vi "Data Viewer.vi"(8 "error in (no error)":errorcluster, 10 "stop pointer":refnum<class "Pointer.lvclass">, 11 "Server IP Address":string="localhost") -> (0 "error out":errorcluster)   [LabVIEW 2017, in "Data Viewer.lvlib"]
uses:
  Core/VIs/Data Viewer/Source/Data Viewer.lvlib
  <vilib>/NI/Memory Manager/Classes/Pointer/Pointer.lvclass
  Main VI/Application Data.ctl
  Buffer Reader/Queue Data.ctl
  Buffer Reader/Buffer Data.ctl
  Core/Classes/Configuration/Core/Transfer/Channel Configuration.ctl
  Core/Typedefs/Core Channel Configuration.ctl
  Core/Typedefs/DSF Data Type.ctl
  Core/Typedefs/DSF Settings Info.ctl
  Core/Typedefs/DSF Byte Order.ctl
  Core/Classes/Thread/Data Server/DSF Buffer Subset Descriptor.ctl
  Core/Typedefs/DSF Buffer Type.ctl
  Main VI/Values Channels.ctl
  Core/Classes/Configuration/Core/Framework/Framework Configuration.lvclass
  <vilib>/NI/Memory Manager/Classes/Pointer/Pointer.lvclass/Pointer.ctl
  <vilib>/NI/Memory Manager/Classes/Pointer/Write Bool.vi
  <vilib>/NI/Memory Manager/Classes/Pointer/Read Bool.vi
  <vilib>/NI/Memory Manager/Classes/Pointer/Get Address.vi
  <vilib>/NI/Memory Manager/Classes/Pointer/Set Address.vi
  <vilib>/NI/Memory Manager/Classes/Pointer/Set Size.vi
  <vilib>/NI/Memory Manager/Classes/Pointer/Set Internal.vi
  <vilib>/NI/Memory Manager/Classes/Pointer/Write (No Check).vi
  <vilib>/NI/Memory Manager/Classes/Pointer/Write (No Check) Bool.vi
  <vilib>/NI/Memory Manager/Classes/Pointer/Check Move.vi
  <vilib>/NI/Memory Manager/Classes/Pointer/Read (No Check).vi
  <vilib>/NI/Memory Manager/Classes/Pointer/Read (No Check) Bool.vi
  <vilib>/NI/Memory Manager/Classes/Pointer/Check Null Pointer.vi
  <vilib>/NI/Memory Manager/Classes/Pointer/Check Count.vi
  <vilib>/NI/Memory Manager/Classes/Pointer/Check Bounds (Power of 2).vi
  <vilib>/NI/Memory Manager/Classes/Pointer/Errors.vi
  <vilib>/NI/Memory Manager/Classes/Pointer/Null Pointer.vi
  <vilib>/NI/Memory Manager/Classes/Pointer/Get Size.vi
  <vilib>/NI/Memory Manager/Classes/Pointer/Out of Bounds.vi
  <vilib>/NI/Memory Manager/Classes/Pointer/Check Bounds.vi
  <vilib>/NI/Memory Manager/Classes/Pointer/Create Error.vi
  <vilib>/NI/Memory Manager/VIs/Write String to Source.vi
  <vilib>/NI/Memory Manager/Classes/Pointer/Write Pointer Size to Error.vi
  <vilib>/NI/Memory Manager/VIs/Write Numeric to Source.vi
  <vilib>/NI/Memory Manager/VIs/Write Numeric Scalar to Source (Base10 U64).vi
  <vilib>/NI/Memory Manager/Classes/Pointer/Check Bounds (Pointer).vi
  <vilib>/NI/Memory Manager/Classes/Pointer/Check Bounds (Buffer).vi
  <vilib>/NI/Memory Manager/VIs/New Error Cluster.vi
  <vilib>/NI/Memory Manager/VIs/New Error Cluster (512B).vi
  <vilib>/NI/Memory Manager/VIs/Set Error Status.vi
  <vilib>/NI/Memory Manager/VIs/Set Error Code.vi
  <vilib>/NI/Memory Manager/VIs/Set Error Source.vi
  <vilib>/NI/Memory Manager/Constants/Constants.vi
  <vilib>/NI/Memory Manager/Constants/Library Name.vi
  <vilib>/NI/Memory Manager/Classes/Pointer/Pointer Error Info.vi
  <vilib>/NI/Memory Manager/Constants/Pointer Class Name.vi
  <vilib>/NI/Memory Manager/Classes/Pointer/Buffer Underflow.vi
  Core/DSF Core.lvlib
  Core/Classes/Configuration/Core/Channel/Channel Configuration.lvclass
  Core/Classes/Configuration/Core/Transfer/Transfer Configuration.lvclass
panel:
  in  "Connect":bool
  out "Connected":bool
  in  "Item Tree":string(tree)
  out "Duration":u64 format="%d µs"
  out "Values":string
  out "ASCII":string
  out "Late Count":u64
  out "Iteration":u64
  out "Frequency":dbl format="%.1fHz"
  out "Size":u64 format="%dB"
  out "Decimation":u64
  out "Throughput":dbl format="%_3pB/s"
  out "Hex":string
  # "Data Viewer"
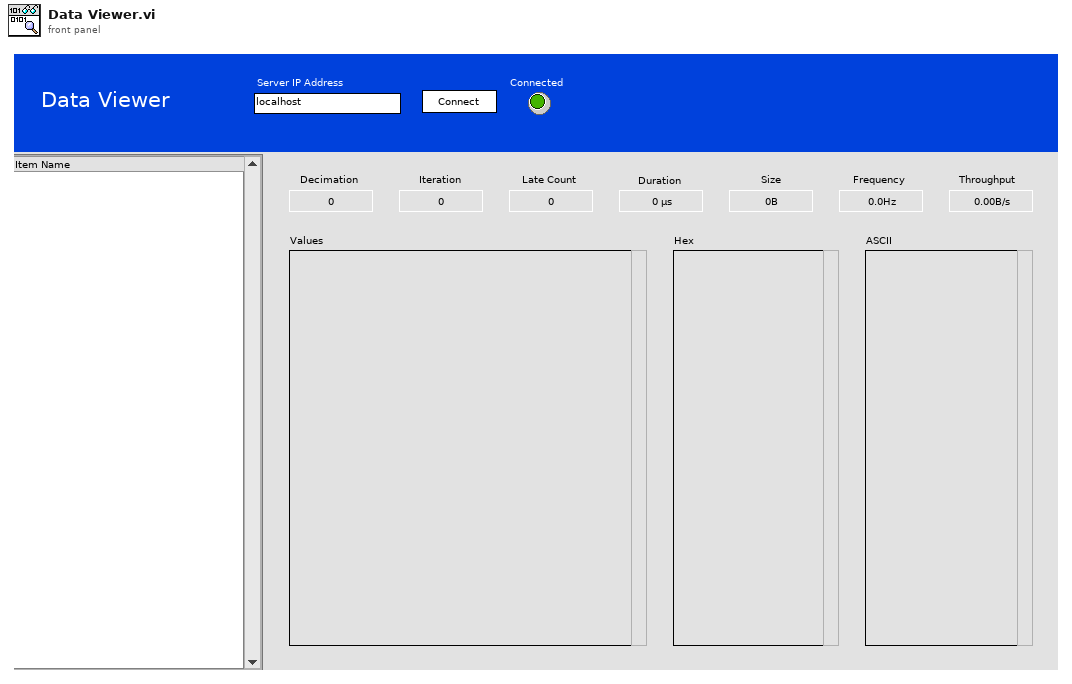
[diagram p1: front panel]
types:
  T1 = typedef "Data Viewer.lvlib/Queue Data.ctl" = cluster{"server ID":refnum<k5>, "Buffer data":T2}
  T2 = typedef "Data Viewer.lvlib/Buffer Data.ctl" = cluster{"decimation":u64, "avg bandwidth":dbl, "channels":T3[], "byte order":T7, "buffer descriptor":T8, "values channels":T10, "select start offset":u64, "select end offset":u64, "channel index":i32}
  T3 = typedef "DSF Core.lvlib/Transfer Configuration.lvclass/Channel Configuration.ctl" = cluster{"configuration":T4, "component settings":T6[]}
  T4 = typedef "DSF Core.lvlib/Channel Configuration.lvclass/Core Channel Configuration.ctl" = cluster{"name":string, "units":string, "engine data type":T5, "string data type":T5, "string offset":u64}
  T5 = typedef "DSF Core.lvlib/DSF Data Type.ctl" = enum8{"Bool", "SGL", "DBL", "I8", "I16", "I32", "I64", "U8", "U16", "U32", "U64"}
  T6 = typedef "DSF Core.lvlib/DSF Settings Info.ctl" = cluster{"component":string, "values":cluster{"key":string, "value":string}[]}
  T7 = typedef "DSF Core.lvlib/DSF Byte Order.ctl" = enum8{"big-endian", "little-endian"}
  T8 = typedef "DSF Core.lvlib/DSF Buffer Subset Descriptor.ctl" = cluster{"buffer type":T9, "plugin id":i32, "group id":i32, "transfer id":i32, "offset":u64, "length":i64}
  T9 = typedef "DSF Core.lvlib/DSF Buffer Type.ctl" = enum16{"Engine", "String"}
  T10 = typedef "Data Viewer.lvlib/Values Channels.ctl" = cluster{"index":i32, "count":i32, "engine offset":u64}
  T11 = typedef "Data Viewer.lvlib/Application Data.ctl" = cluster{"Item Tree Control":refnum<vi>, "Top-Level VI":refnum<vi>, "menu reference":refnum<k9>, "queue":refnum<queue>, "Stop Pointer":refnum<class "Pointer.lvclass">, "Buffer Variant":variant, "server ID":refnum<k5>, "framework tag":string, "Values":refnum<vi>, "Hex":refnum<vi>, "ASCII":refnum<vi>, "lines visible":i32, "values padding":i32, "current buffer data":T2, "Framework Configuration":refnum<class "Framework Configuration.lvclass">}
  T12 = typedef "LVPoint32TypeDef.ctl" = cluster{"Horizontal":i32, "Vertical":i32}
  T13 = typedef "DSF Core.lvlib/DSF Performance Metrics.ctl" = cluster{"framework period":u32, "iteration":u64, "late count":u64, "duration":u64}
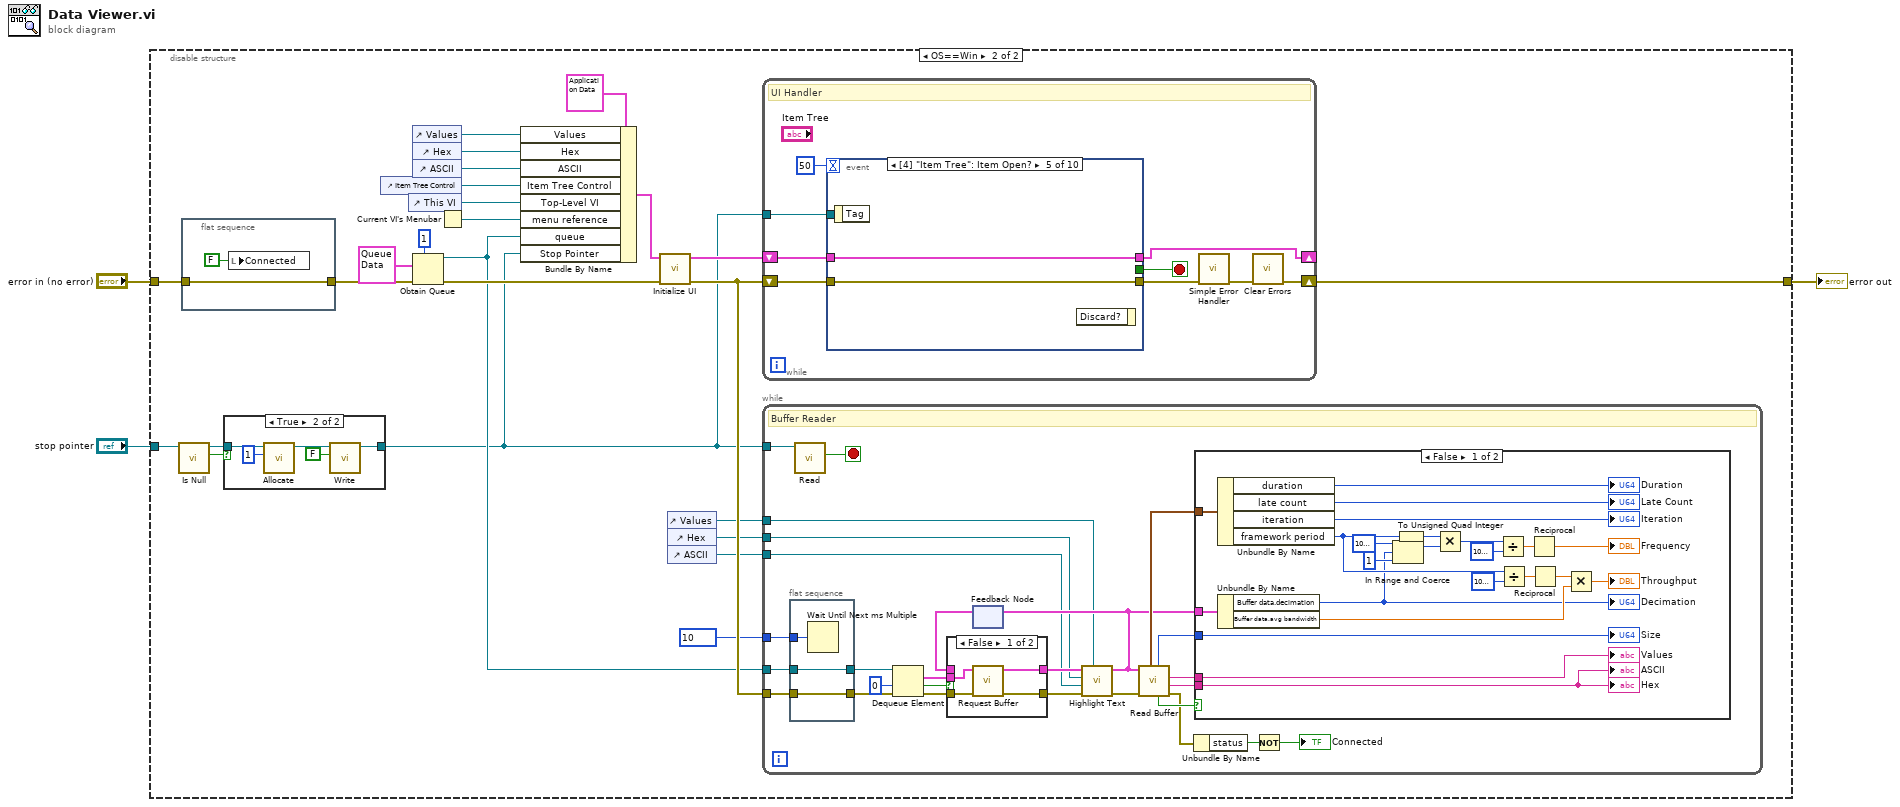
[diagram p0: block diagram]
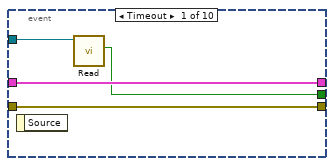
[diagram p6: hidden frame]
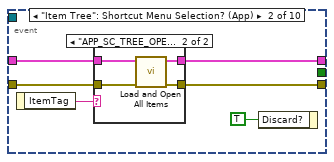
[diagram p7: hidden frame]
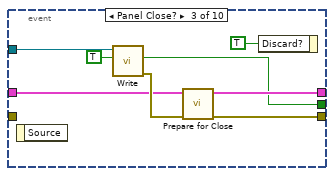
[diagram p9: hidden frame]
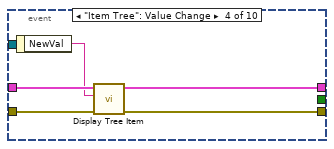
[diagram p10: hidden frame]
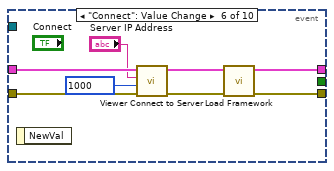
[diagram p11: hidden frame]
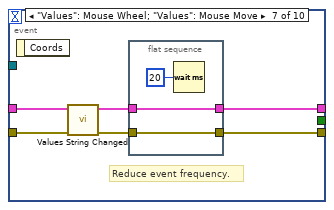
[diagram p12: hidden frame]
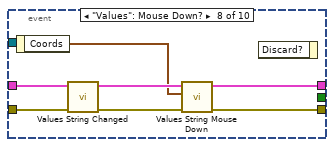
[diagram p13: hidden frame]
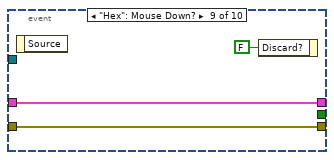
[diagram p14: hidden frame]
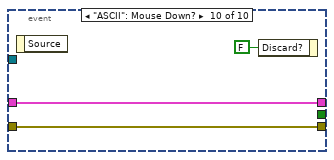
[diagram p15: hidden frame]
diagram:
  n1 = disable-structure shown="OS==Win" {
    disable-tunnel: "error in (no error)" -> [w4 w28]
    disable-tunnel: "stop pointer" -> [_ w27]
    disable-tunnel: [w4 w26] -> w1
    frame condition #0 {
    }
    frame condition #1 (active) {
      n2 = call <vilib>:"Is Null.vi"("Pointer in"=w27) -> ("null?"=w18:bool)  [unwired: 8 in, 2 out]
      n3 = flat-sequence {
        tunnel: [w29] -> w13
        tunnel: w28 -> [w29]
        frame #0 {
          n4 = local write "Connected"(FALSE ("Connected")) -> ()
        }
      }
      n5 = case shown="True" w18 {
        tunnel: [w31 w33] -> w12
        tunnel: w27 -> [w31 w35]
        frame False {
        }
        frame True {
          n6 = call <vilib>:"Allocate.vi"("size"=u64 1, "Pointer type"=w35) -> ("Pointer out"=w34:refnum<class "Pointer.lvclass">)  [unwired: 8 in, 1 out]
          n7 = call-poly <vilib>:"Write.vi"("value"=FALSE ("buffer in"), "Pointer in"=w34) -> ("Pointer out"=w33:refnum<class "Pointer.lvclass">)  [unwired: 6 in, 3 out]
        }
      }
      n8 = control-ref of="Item Tree Control"() -> (w22:refnum<vi>)
      n9 = control-ref of="This VI"() -> (w24:refnum<vi>)
      n10 = control-ref of="Values"() -> (w8:refnum<vi>)
      n11 = control-ref of="Hex"() -> (w9:refnum<vi>)
      n12 = control-ref of="ASCII"() -> (w10:refnum<vi>)
      n13 = Obtain Queue(max queue size (-1, unlimited)=1, element data type=T1 {"server ID"=refnum, "Buffer data"={"decimation"=0, "avg bandwidth"=0.0, "channels"=[], "byte order"=enum."little-endian", "buffer descriptor"={"buffer type"=enum."Engine", "plugin id"=0, "group id"=0, "transfer id"=0, "offset"=0, "length"=0}, "values channels"={"index"=0, "count"=0, "engine offset"=0}, "select start offset"=18446744073709551615, "select end offset"=0, "channel index"=-1}} ("Queue data"), error in (no error)=w13) -> (queue out=w14:refnum<queue>, error out=w21:errorcluster)  [unwired: 2 in, 1 out]
      n14 = Current VI's Menubar() -> (w23:refnum<k9>)
      n15 = Bundle By Name(cluster=T11 {"Item Tree Control"=refnum, "Top-Level VI"=refnum, "menu reference"=refnum, "queue"=refnum, "Stop Pointer"=refnum, "Buffer Variant"=variant, "server ID"=refnum, "framework tag"="", "Values"=refnum, "Hex"=refnum, "ASCII"=refnum, "lines visible"=0, "values padding"=0, "current buffer data"={"decimation"=0, "avg bandwidth"=0.0, "channels"=[], "byte order"=enum."big-endian", "buffer descriptor"={"buffer type"=enum."Engine", "plugin id"=0, "group id"=0, "transfer id"=0, "offset"=0, "length"=0}, "values channels"={"index"=0, "count"=0, "engine offset"=0}, "select start offset"=0, "select end offset"=0, "channel index"=0}, "Framework Configuration"=refnum}, "Values"=w8, "Hex"=w9, "ASCII"=w10, "Item Tree Control"=w22, "Top-Level VI"=w24, "menu reference"=w23, "queue"=w14, "Stop Pointer"=w12) -> (w17:T11)
      n16 = call "Initialize UI.vi"("error in (no error)"=w21, "Application Data in"=w17) -> ("error out"=w16:errorcluster, "Application Data out"=w20:T11)  [unwired: 8 in]
      n17 = control-ref of="Values"() -> (w5:refnum<vi>)
      n18 = control-ref of="Hex"() -> (w6:refnum<vi>)
      n19 = control-ref of="ASCII"() -> (w7:refnum<vi>)
      n20 = while {
        shift-right: [w96] -> w26
        shift-left: w16 -> [w104]
        shift-right: [w101] -> _
        shift-left: w20 -> [w100]
        tunnel: w12 -> [w98]
        stop <- w99 stop-if-true
        # "UI Handler"
        n21 = event shown="[4] \"Item Tree\": Item Open?" {
          selector: _ -> [_ _ _ _ _ _ _ _ _ _]
          dyn-events: _ -> [_ _ _ _ _ _ _ _ _ _]
          timeout: 50 -> [_ _ _ _ _ _ _ _ _ _]
          tunnel: [w105 _ w123 _ _ _ _ _ _ _] -> w99
          tunnel: w104 -> [w108 w111 _ w133 w135 w142 w149 w158 w162 w165]
          tunnel: [w108 w112 w127 w132 w135 w137 w146 w154 w162 w165] -> w102
          tunnel: w100 -> [w107 w113 w121 w130 w134 w143 w148 w159 w161 w164]
          tunnel: [w107 w109 w126 w131 w134 w136 w144 w155 w161 w164] -> w101
          tunnel: w98 -> [w106 _ w125 _ _ _ _ _ _ _]
          event Timeout {
            n22 = event-data() -> ()  [unwired: 1 in, 1 out]
            n23 = call-poly <vilib>:"Read.vi"("Pointer in"=w106) -> ("value out"=w105:bool)  [unwired: 7 in, 3 out]
          }
          event "Item Tree": Shortcut Menu Selection? (App) {
            n24 = event-data() -> ("ItemTag"=w114:string)  [unwired: 1 in]
            n25 = case shown="\"APP_SC_TREE_OPEN_ALL_ITEMS\"" w114 {
              tunnel: w113 -> [w115 w120]
              tunnel: [w116 w118] -> w112
              tunnel: w111 -> [w116 w119]
              tunnel: [w115 w117] -> w109
              frame Default {
              }
              frame "APP_SC_TREE_OPEN_ALL_ITEMS" {
                n26 = call "Load and Open All Items.vi"("error in (no error)"=w119, "Application Data in"=w120) -> ("error out"=w118:errorcluster, "Application Data out"=w117:T11)  [unwired: 8 in]
              }
            }
            n27 = event-data("Discard?"=TRUE) -> ()  [unwired: 1 in, 1 out]
          }
          event Panel Close? {
            n28 = event-data() -> ()  [unwired: 1 in, 1 out]
            n29 = call-poly <vilib>:"Write.vi"("value"=TRUE, "Pointer in"=w125) -> ("error out"=w122:errorcluster, "value"=w123:bool)  [unwired: 6 in, 2 out]
            n30 = call "Prepare for Close.vi"("error in (no error)"=w122, "Application Data in"=w121) -> ("error out"=w127:errorcluster, "Application Data out"=w126:T11)  [unwired: 8 in]
            n31 = event-data("Discard?"=TRUE) -> ()  [unwired: 1 in, 1 out]
          }
          event "Item Tree": Value Change {
            n32 = event-data() -> ("NewVal"=w129:string)  [unwired: 1 in]
            n33 = call "Display Tree Item.vi"("error in (no error)"=w133, "Tag"=w129, "Application Data in"=w130) -> ("error out"=w132:errorcluster, "Application Data out"=w131:T11)  [unwired: 7 in]
          }
          event "Item Tree": Item Open? {
            n34 = event-data() -> ()  [unwired: 1 in, 1 out]
            n35 = event-data() -> ()  [unwired: 2 in, 1 out]
          }
          event "Connect": Value Change {
            n36 = event-data() -> ()  [unwired: 1 in, 1 out]
            n37 = call "Viewer Connect to Server.vi"("error in (no error)"=w142, "timeout ms (60000)"=1000, "server address"="Server IP Address", "Application Refs"=w143) -> ("error out"=w138:errorcluster, "Application Data out"=w139:T11)  [unwired: 6 in]
            n38 = call "Load Framework.vi"("error in (no error)"=w138, "Application Refs"=w139) -> ("error out"=w137:errorcluster, "Application Data out"=w136:T11)  [unwired: 8 in]
          }
          event "Values": Mouse Wheel; "Values": Mouse Move {
            # "Reduce event frequency."
            n39 = event-data() -> ()  [unwired: 1 in, 1 out]
            n40 = call "Values String Changed.vi"("error in (no error)"=w149, "Application Data in"=w148) -> ("error out"=w147:errorcluster, "Application Data out"=w145:T11)  [unwired: 8 in]
            n41 = flat-sequence {
              tunnel: w147 -> [w151]
              tunnel: [w151] -> w146
              tunnel: w145 -> [w150]
              tunnel: [w150] -> w144
              frame #0 {
                n42 = Wait (ms)(milliseconds to wait=u32 20) -> ()  [unwired: 1 out]
              }
            }
          }
          event "Values": Mouse Down? {
            n43 = event-data() -> ("Coords"=w153:T12)  [unwired: 1 in]
            n44 = call "Values String Changed.vi"("error in (no error)"=w158, "Application Data in"=w159) -> ("error out"=w156:errorcluster, "Application Data out"=w157:T11)  [unwired: 8 in]
            n45 = call "Values String Mouse Down.vi"("error in (no error)"=w156, "Coords"=w153, "Application Data in"=w157) -> ("error out"=w154:errorcluster, "Application Data out"=w155:T11)  [unwired: 7 in]
            n46 = event-data() -> ()  [unwired: 2 in, 1 out]
          }
          event "Hex": Mouse Down? {
            n47 = event-data() -> ()  [unwired: 1 in, 1 out]
            n48 = event-data("Discard?"=FALSE) -> ()  [unwired: 1 in, 1 out]
          }
          event "ASCII": Mouse Down? {
            n49 = event-data() -> ()  [unwired: 1 in, 1 out]
            n50 = event-data("Discard?"=FALSE) -> ()  [unwired: 1 in, 1 out]
          }
        }
        n51 = call <vilib>:"Simple Error Handler.vi"("error in (no error)"=w102) -> ("error out"=w103:errorcluster)  [unwired: 4 in, 4 out]
        n52 = call <vilib>:"Clear Errors.vi"("error in (no error)"=w103) -> ("error out"=w96:errorcluster)  [unwired: 5 in, 1 out]
      }
      n53 = while {
        tunnel: w14 -> [w50]
        tunnel: w12 -> [w61]
        tunnel: w16 -> [w49]
        tunnel: u32 10 ("milliseconds to wait") -> [w46]
        tunnel: w7 -> [w37]
        tunnel: w6 -> [w40]
        tunnel: w5 -> [w39]
        stop <- w62 stop-if-true
        # "Buffer Reader"
        n54 = flat-sequence {
          tunnel: w50 -> [w65]
          tunnel: w49 -> [w66]
          tunnel: [w66] -> w47
          tunnel: [w65] -> w48
          tunnel: w46 -> [w64]
          frame #0 {
            n55 = Wait Until Next ms Multiple(millisecond multiple=w64) -> ()  [unwired: 1 out]
          }
        }
        n56 = call-poly <vilib>:"Read.vi"("Pointer in"=w61) -> ("value out"=w62:bool)  [unwired: 7 in, 3 out]
        n57 = Dequeue Element(queue=w48, timeout in ms (-1)=0, error in (no error)=w47) -> (element=w57:T1, timed out?=w56:bool, error out=w58:errorcluster)  [unwired: 1 out]
        n58 = feedback #1() -> (w55:T1)  [unwired: 1 in]
        n59 = case shown="False" w56 {
          tunnel: w58 -> [w70 w71]
          tunnel: w57 -> [w69 _]
          tunnel: [w68 w71] -> w44
          tunnel: [w67 w72] -> w43
          tunnel: w55 -> [_ w72]
          frame False {
            n60 = call "Request Buffer.vi"("error in (no error)"=w70, "queue data in"=w69) -> ("error out"=w68:errorcluster, "queue data out"=w67:T1)  [unwired: 8 in]
          }
          frame True {
          }
        }
        n61 = call "Highlight Text.vi"("Values"=w39, "error in (no error)"=w44, "ASCII"=w37, "Hex"=w40, "queue data in"=w43) -> ("error out"=w42:errorcluster, "queue data out"=w41:T1)  [unwired: 5 in]
        n62 = feedback-in #1(w41) -> ()
        n63 = call "Read Buffer.vi"("error in (no error)"=w42, "queue data in"=w41) -> ("error out"=w38:errorcluster, "buffer data"=w59:string, "values string"=w45:string, "timed out?"=w53:bool, "buffer size"=w60:u64, "metrics"=w51:T13)  [unwired: 3 in, 1 out]
        n64 = Unbundle By Name(w38) -> ("status"=w54:bool)
        n65 = case shown="False" w53 {
          tunnel: w60 -> [w85 _]
          tunnel: w45 -> [w84 _]
          tunnel: w59 -> [w83 _]
          tunnel: w51 -> [w79 _]
          tunnel: w41 -> [w78 _]
          frame False {
            n66 = Unbundle By Name(w79) -> ("duration"=→"Duration":u64, "late count"=→"Late Count":u64, "iteration"=→"Iteration":u64, "framework period"=w74:u32)
            n67 = Unbundle By Name(w78) -> ("Buffer data.decimation"=w73:u64, "Buffer data.avg bandwidth"=w80:dbl)
            "Decimation" <- w73
            n68 = In Range and Coerce(upper limit=u64 1000000 ("lower limit"), x=w73, lower limit=u64 1) -> (coerced(x)=w89:u64)  [unwired: 1 out]
            n69 = To Unsigned Quad Integer(1:w74) -> (0:w92:u64)
            n70 = Multiply(x=w92, y=w89) -> (x*y=w95:u64)
            n71 = Divide(x=w95, y=u64 1000000) -> (x/y=w91:dbl)
            n72 = Divide(x=w74, y=u64 1000000) -> (x/y=w87:dbl)
            n73 = Reciprocal(x=w91) -> (1/x=→"Frequency":dbl)
            n74 = Reciprocal(x=w87) -> (1/x=w86:dbl)
            n75 = Multiply(x=w86, y=w80) -> (x*y=→"Throughput":dbl)
            "Hex" <- w83
            "Size" <- w85
            "ASCII" <- w83
            "Values" <- w84
          }
          frame True {
          }
        }
        n76 = Not(x=w54) -> (.not. x?=→"Connected":bool)
      }
    }
  }
  "error out" <- w1
